vi "MH_CalcBinningValues.vi"(10 "BaseResolution":u32=10, 11 "Bin Steps":i32) -> (3 "BinningValues":cluster{"String":string, "Value":i32}[](array[cluster]))   [LabVIEW 2019]
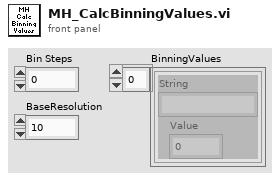
[diagram p1: front panel]
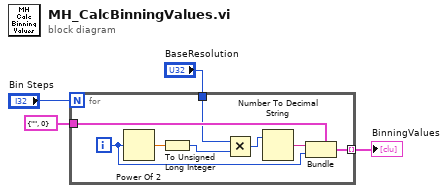
[diagram p0: block diagram]
diagram:
  n1 = for {
    N: "Bin Steps" -> [_]
    tunnel: cluster{"String":string, "Value":i32} {"String"="", "Value"=0} -> [w12]
    tunnel: [w6] -> w4 mode=indexing
    tunnel: "BaseResolution" -> [w5]
    i -> [w11]
    n2 = Power Of 2(x=w11) -> (2^x=w10:dbl)
    n3 = To Unsigned Long Integer(number=w10) -> (unsigned 32bit integer=w9:u32)
    n4 = Multiply(x=w5, y=w9) -> (x*y=w8:u32)
    n5 = Number To Decimal String(number=w8) -> (decimal integer string=w7:string)  [unwired: 1 in]
    n6 = Bundle(cluster=w12, "String"=w7, "Value"=w11) -> (w6:cluster{"String":string, "Value":i32})
  }
  "BinningValues" <- w4
